vi "Deserialize_To_Same.vi"(8 "error in (no error)":errorcluster, 10 "To Object":refnum<class>, 11 "From Object":refnum<class>) -> (0 "error out":errorcluster, 3 "Target Object":refnum<class>)   [LabVIEW 2020, in "BlueSerialization.lvlib" / "BlueSerializer.lvclass"]
uses:
  BlueSerializer.lvclass
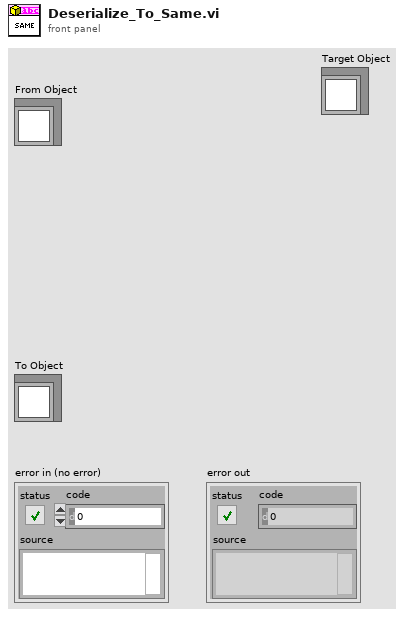
[diagram p1: front panel]
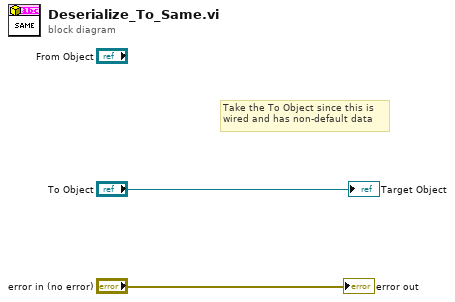
[diagram p0: block diagram]
diagram:
  # "Take the To Object since this is\nwired and has non-default data"
  "error out" <- "error in (no error)"
  "Target Object" <- "To Object"
